vi "TempVI Attempt.vi"(8 "error in (no error)":errorcluster, 11 "notifier":refnum<notifier>) -> (0 "error out":errorcluster, 3 "Mean":sgl)   [LabVIEW 2014]
panel:
  in  "Reset Data Analysis":bool
  out "Total Samples":sgl
  out "Min":sgl
  out "Max":sgl
  out "Standard Dev":sgl
  in  "Number of Samples":u32=600
  out "Waveform Chart":dynamicdata(graph)
  in  "Delay Time (s)":sgl=1.0
  in  "?":bool
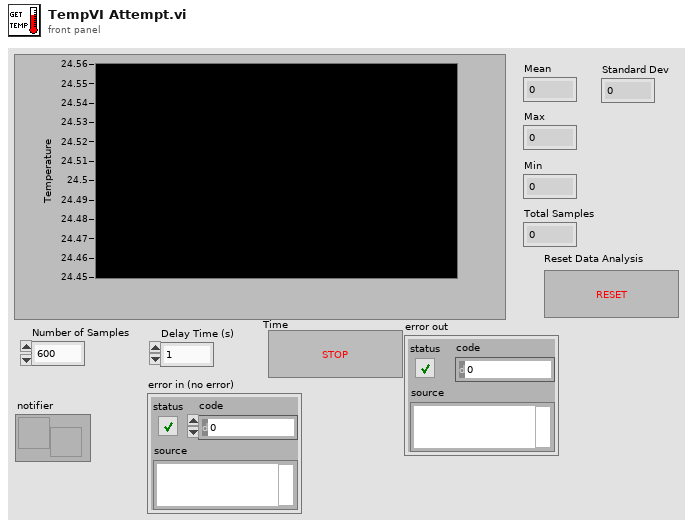
[diagram p1: front panel]
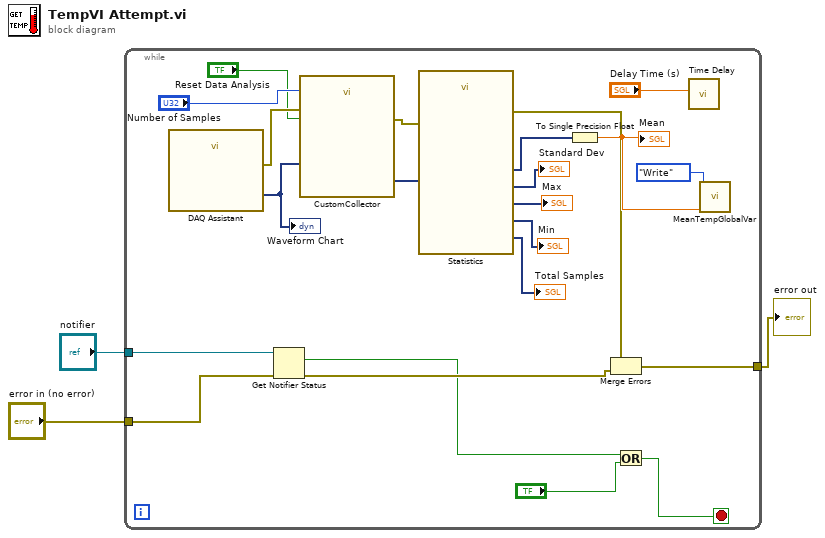
[diagram p0: block diagram]
diagram:
  n1 = while {
    tunnel: "notifier" -> [w11]
    tunnel: "error in (no error)" -> [w10]
    tunnel: [w7] -> w1
    stop <- w4 stop-if-true
    n2 = call "DAQ Assistant"() -> ("data"=w24:dynamicdata, "error out"=w22:errorcluster)  [unwired: 17 in, 1 out]
    "Waveform Chart" <- w24
    n3 = Get Notifier Status(notifier=w11, error in (no error)=w10) -> (current notification=w5:bool, error out=w8:errorcluster)  [unwired: 3 out]
    n4 = call "CustomCollector.vi"("Reset"="Reset Data Analysis", "error in (no error)"=w22, "Size"="Number of Samples", "Signals"=w24) -> ("error out"=w21:errorcluster, "Collected Signals"=w23:dynamicdata)  [unwired: 6 in]
    n5 = call "Statistics"("Signals"=w23, "error in (no error)"=w21) -> ("Total Samples"=→"Total Samples":dynamicdata, "Standard Dev"=→"Standard Dev":dynamicdata, "Arithmetic Mean"=w14:dynamicdata, "Minimum"=→"Min":dynamicdata, "Maximum"=→"Max":dynamicdata, "error out"=w9:errorcluster)  [unwired: 20 in]
    n6 = To Single Precision Float(number=w14) -> (single precision float=w12:sgl)
    "Mean" <- w12
    n7 = Merge Errors(w9, w8) -> (w7:errorcluster)
    n8 = Or(x=w5, y="?") -> (x .or. y?=w4:bool)
    n9 = call "Time Delay"("Delay Time (s)"="Delay Time (s)") -> ()  [unwired: 10 in, 1 out]
    n10 = call "MeanTempGlobalVar.vi"("Temp In"=w12, "State"=enum16{"Initialise", "Write", "Read"}."Write") -> ()  [unwired: 9 in, 1 out]
  }
  "error out" <- w1
